vi "Insert Image (ARGB).vi"(7 "Offset (Default: 0,0)":T1, 8 "error in (no error)":errorcluster, 9 "ARGB Image Destination in":T2, 10 "ARGB Image Child in":T2, 11 "ARGB Image Parent in":T2) -> (0 "error out":errorcluster, 3 "ARGB Image Destination":T2)   [LabVIEW 2020, in "image.lvlib"]
doc: "Copy the the Child Image over the Parent Image with the given offset."
uses:
  image.lvlib
  ARGB Image.ctl
  common/Image Point (Integer).ctl
  5e3288c8-ee88-4cfe-89cf-31ceca475f5a.vi
  <vilib>/Utility/error.llb/Error Cluster From Error Code.vi
  common/common.lvlib
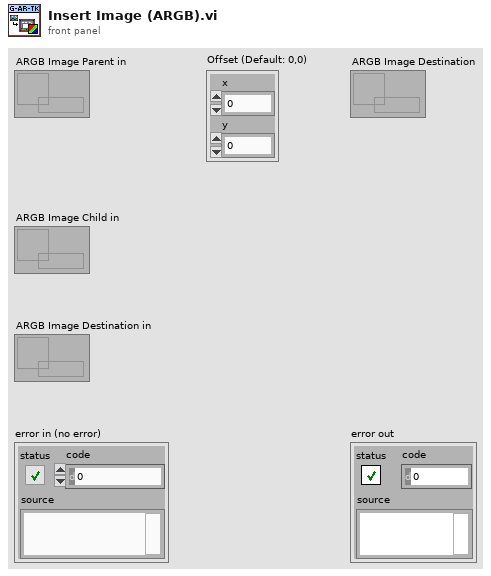
[diagram p1: front panel]
types:
  T1 = typedef "common.lvlib/Image Point (Integer).ctl" = cluster{"x":i32, "y":i32}
  T2 = typedef "image.lvlib/ARGB Image.ctl" = refnum<data-value>
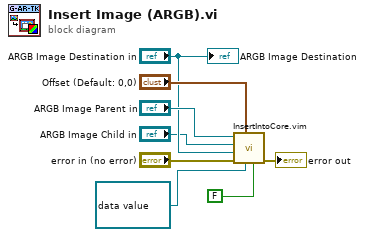
[diagram p0: block diagram]
diagram:
  n1 = call "InsertIntoCore.vim"("Has Mask"=FALSE, "Mask"=refnum<data-value> refnum, "Offset"="Offset (Default: 0,0)", "error in (no error)"="error in (no error)", "Dst"="ARGB Image Destination in", "Src_Child"="ARGB Image Child in", "Src_Parent"="ARGB Image Parent in") -> ("error out"=→"error out":errorcluster)  [unwired: 4 in]
  "ARGB Image Destination" <- "ARGB Image Destination in"
